vi "Get Bitfile Property Name.vi"(11 "RIO Device Address in":string) -> (3 "Bitfile Property Name":string)   [LabVIEW 2017, in "Engine Simulation Toolkit System Explorer.lvlib"]
uses:
  Engine Simulation Toolkit System Explorer.lvlib
  Shared/Properties.vi
  Shared/Engine Simulation Toolkit Shared.lvlib
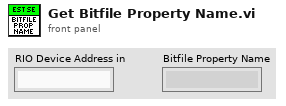
[diagram p1: front panel]
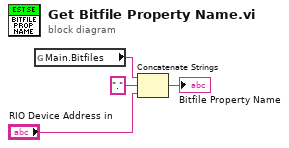
[diagram p0: block diagram]
diagram:
  n1 = global read "Properties.vi" "Main.Bitfiles"() -> (w4:string)
  n2 = Concatenate Strings(w4, "." ("string"), "RIO Device Address in") -> (→"Bitfile Property Name":string)
